vi "SetHorizontal.vi"(8 "error in (no error)":errorcluster, 10 "Horizontal Settings":T2={"Time/div"=0.01, "Trigger Holdoff"=0.0} {"Time/div" scale=0.0001..1.0 scale format="%#_8g"}, 11 "reference in":refnum<k24>) -> (0 "error out":errorcluster, 1 "Setup Info Horizontal":T1, 3 "reference out":refnum<k24>)   [LabVIEW 2019, in "LabNation Scope Driver.lvlib"]
uses:
  LabNation Scope Driver.lvlib
  C:/Program Files (x86)/LabNation/SmartScope/DeviceInterface.dll
  Program Files (x86)/LabNation/SmartScope/DeviceInterface.dll
  Typedef/Horizontal Settings.ctl
  Typedef/TimeSetting.ctl
  Typedef/Setup Info Horizontal.ctl
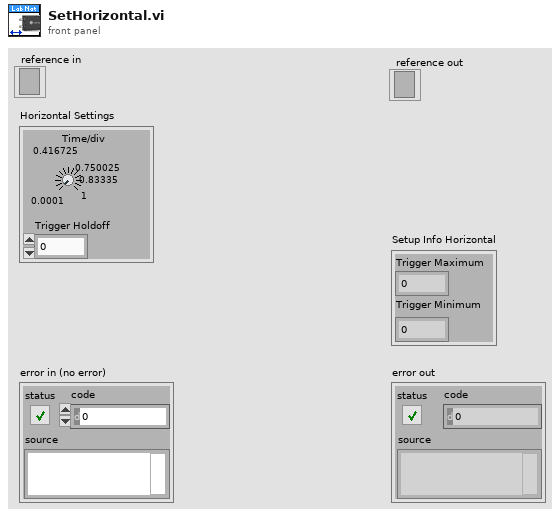
[diagram p1: front panel]
types:
  T1 = typedef "LabNation Scope Driver.lvlib/Setup Info Horizontal.ctl" = cluster{"Trigger Maximum":dbl, "Trigger Minimum":dbl}
  T2 = typedef "LabNation Scope Driver.lvlib/Horizontal Settings.ctl" = cluster{"Time/div":T3, "Trigger Holdoff":dbl}
  T3 = typedef "LabNation Scope Driver.lvlib/TimeSetting.ctl" = dbl
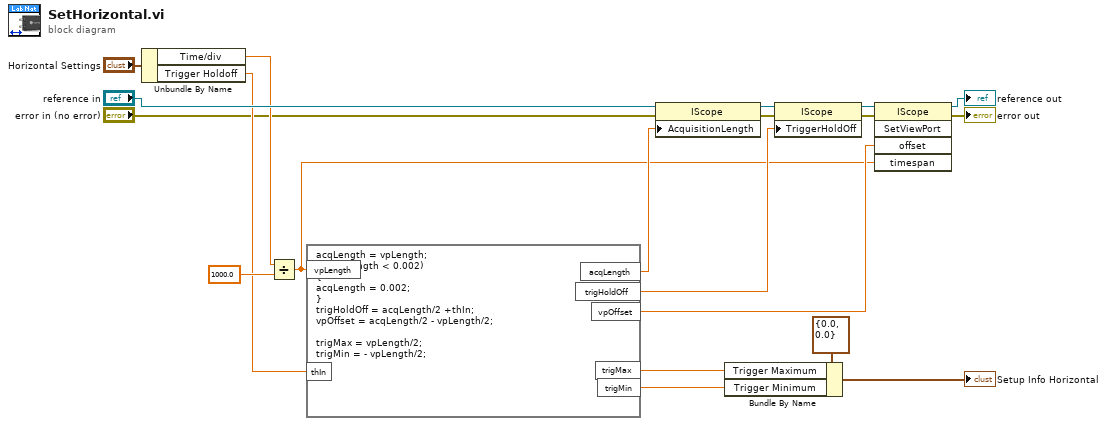
[diagram p0: block diagram]
diagram:
  n1 = Unbundle By Name("Horizontal Settings") -> ("Time/div"=w10:T3, "Trigger Holdoff"=w8:dbl)
  n2 = Divide(x=w10, y=1000.0) -> (x/y=w9:T3)
  n3 = formula code="acqLength = vpLength;\nif (acqLength < 0.002)\n{\nacqLength = 0.002;\n}\ntrigHoldOff = acqLength/2 +thIn;\nvpOffset = acqLength/2 - vpLength/2;\n\ntrigMax = vpLength/2;\ntrigMin = - vpLength/2;"("vpLength"=w9, "thIn"=w8) -> ("acqLength"=w17:dbl, "trigHoldOff"=w15:dbl, "vpOffset"=w18:dbl, "trigMax"=w2:dbl, "trigMin"=w1:dbl)
  n4 = property class="IScope"(reference="reference in", error in="error in (no error)", "AcquisitionLength"=w17) -> (reference out=w16:refnum<k24>, error out=w6:errorcluster)
  n5 = Bundle By Name(cluster=T1 {"Trigger Maximum"=0.0, "Trigger Minimum"=0.0} ("Setup Info Horizontal"), "Trigger Maximum"=w2, "Trigger Minimum"=w1) -> (→"Setup Info Horizontal":T1)
  n6 = property class="IScope"(reference=w16, error in=w6, "TriggerHoldOff"=w15) -> (reference out=w19:refnum<k24>, error out=w5:errorcluster)
  n7 = invoke class="IScope" method="SetViewPort"(reference=w19, error in=w5, "offset"=w18, "timespan"=w9) -> (reference out=→"reference out":refnum<k24>, error out=→"error out":errorcluster)  [unwired: 1 in, 3 out]
